vi "DVRtoNumber.vi"(10 "FrameworkDataRef":T1) -> (2 "Number":i32)   [LabVIEW 2016, in "EmbeddedMainUI.lvclass"]
uses:
  EmbeddedMainUI.lvclass
  Typedefs/FrameworkDataRef.ctl
  FrameworkData.ctl
  <vilib>/Levylab/Embedded SMO UI/EmbeddedSMO.lvclass
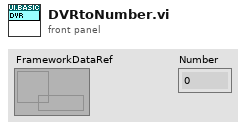
[diagram p1: front panel]
types:
  T1 = typedef "EmbeddedMainUI.lvclass/FrameworkDataRef.ctl" = refnum<data-value>
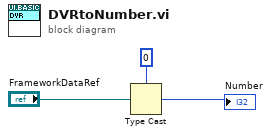
[diagram p0: block diagram]
diagram:
  n1 = Type Cast(type=0, x="FrameworkDataRef") -> (*(type *) &x=→"Number":i32)
